vi "Result_Test.vi"(8 "error in (no error)":errorcluster caption="entrée d'erreur (pas d'erreur)", 11 "Get_Voltage en entrée":refnum<class "P2056_Get_DeviceID.lvclass">) -> (0 "error out":errorcluster caption="sortie d'erreur", 3 "Get_Voltage en sortie":refnum<class "P2056_Get_DeviceID.lvclass">)   [LabVIEW 2020, in "Library Test.lvlib" / "P2056_Get_DeviceID.lvclass"]
uses:
  P2056_Get_DeviceID.lvclass
  C:/Users/ngarcin/OneDrive - Altyor/Standard TB/Suite TB45/Class/Test/Test (Default)/Test (Default).lvclass
  Commun VI/TypeDef/Variable Printable.ctl
  JSON API/JSON Value/Set from JSON string.vi
  JSON API/JSON Value/JSON Value.lvclass
  P2056_Send_Command_UART.lvclass
  JSON API/Variant JSON/Variant JSON.lvlib
  JSON API/Get Polymorphic/JSON GetSet.lvlib
  Commun VI/Library Commun.lvlib
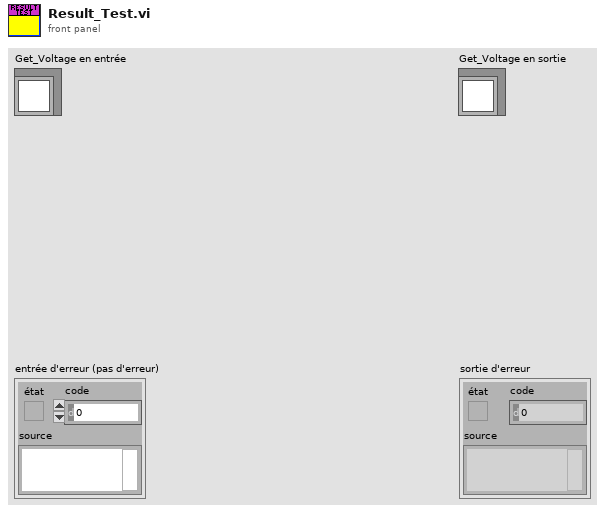
[diagram p1: front panel]
types:
  T1 = typedef "Variable Printable.ctl" = string
  T2 = enum16{"Get Variable", "Get All Variables", "Set Variable", "Delete Variable", "Delete All Variable"}
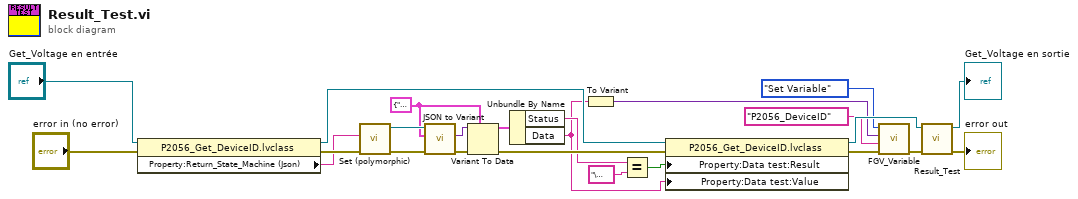
[diagram p0: block diagram]
diagram:
  w17 = cluster{"Data":string, "Status":string} {"Data"="", "Status"=""}
  n1 = property class="P2056_Get_DeviceID.lvclass"(reference="Get_Voltage en entrée", error in="error in (no error)") -> (reference out=w22:refnum<class "P2056_Get_DeviceID.lvclass">, error out=w16:errorcluster, "Property:Return_State_Machine (Json)"=w14:string)
  n2 = call-poly "Set (polymorphic).vi"("error in (no error)"=w16, "JSON stream"=w14) -> ("error out"=w19:errorcluster, "JSON Value out"=w21:refnum<class "JSON Value.lvclass">)  [unwired: 7 in, 1 out]
  n3 = call "JSON to Variant.vi"("error in (no error)"=w19, "Variant (Data Type)"=w17, "JSON Value"=w21) -> ("error out"=w20:errorcluster, "Variant out"=w18:variant)  [unwired: 7 in]
  n4 = Variant To Data(error in=w20, type=w17, Variant=w18) -> (data=w13:cluster{"Data":string, "Status":string}, error out=w15:errorcluster)
  n5 = Unbundle By Name(w13) -> ("Status"=w12:string, "Data"=w2:string)
  n6 = To Variant(anything=w2) -> (Variant=w1:variant)
  n7 = Equal?(x=w12, y="\u0000") -> (x = y?=w10:bool)
  n8 = property class="P2056_Get_DeviceID.lvclass"(reference=w22, error in=w15, "Property:Data test:Result"=w10, "Property:Data test:Value"=w2) -> (reference out=w9:refnum<class "P2056_Get_DeviceID.lvclass">, error out=w4:errorcluster)
  n9 = call "FGV_Variable.vi"("error in (no error)"=w4, "Variable"=T1 "P2056_DeviceID", "Data In"=w1, "Function"=T2."Set Variable") -> ("error out"=w3:errorcluster)  [unwired: 5 in, 2 out]
  n10 = call-parent "Result_Test.vi"("error in (no error)"=w3, "Get_Voltage en entrée"=w9) -> ("error out"=→"error out":errorcluster, "Get_Voltage en sortie"=→"Get_Voltage en sortie":refnum<class "P2056_Get_DeviceID.lvclass">)  [unwired: 8 in]
